vi "utilPlotZeroPole.vi"(3 "a, reverse coefficients":dbl[](array[numeric])=[1.0], 5 "b, forward coefficients":dbl[](array[numeric])) -> (1 "Pole-Zero Plot":cluster{dbl[], dbl[]}[](graph))   [LabVIEW 2016]
doc: "Plot the pole-zero diagram of a filter described by its direct-form \"a\" (reverse) and \"b\" (forward) coefficients."
uses:
  <vilib>/Analysis/1siggen.llb/Ramp Pattern by Samples.vi
  <vilib>/Analysis/polynomials.llb/Remove Zero Coefficients (DBL).vi
  <vilib>/Analysis/polynomials.llb/Polynomial Roots (DBL).vi
  <vilib>/Analysis/NI_AALPro.lvlib
  <vilib>/Analysis/NI_AALBase.lvlib
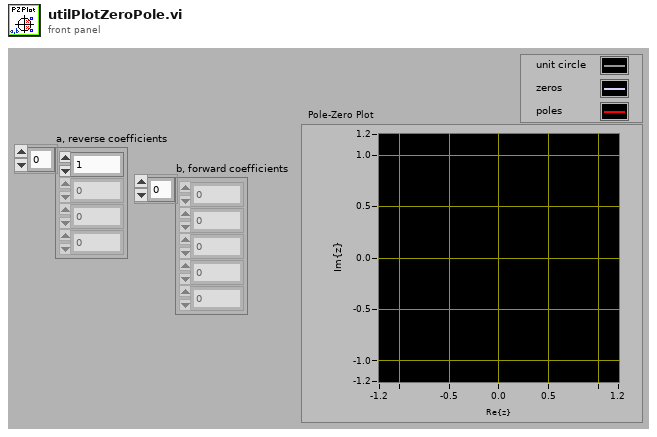
[diagram p1: front panel]
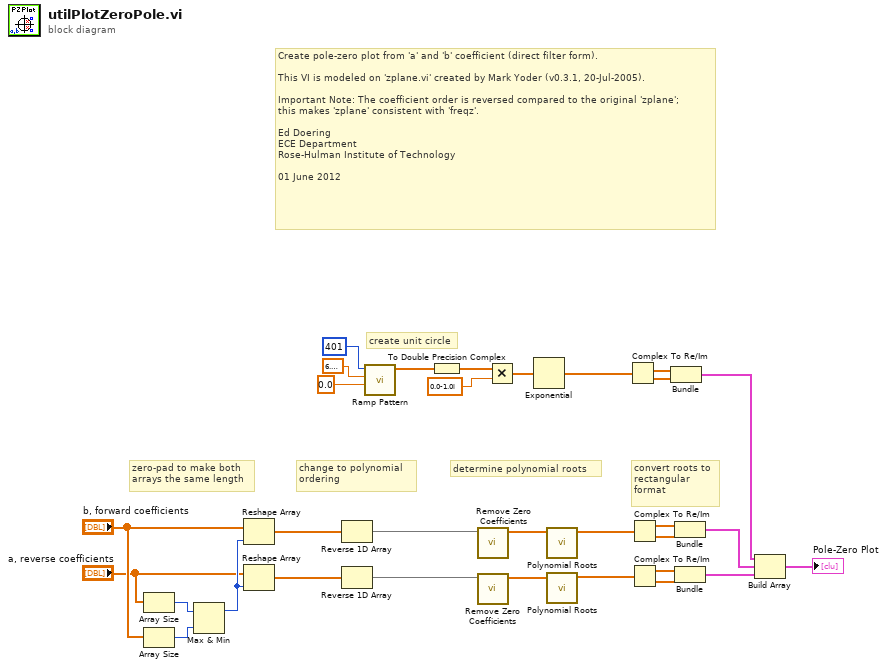
[diagram p0: block diagram]
diagram:
  # "determine polynomial roots"
  # "change to polynomial\nordering"
  # "zero-pad to make both\narrays the same length"
  # "create unit circle"
  # "Create pole-zero plot from 'a' and 'b' coefficient (direct filter form).\n\nThis VI is modeled on 'zplane.vi' created by Mark Yoder (v0.3.1, 20-Jul-2005).\n\nImportant Note: The coefficient order is reversed compared to the original 'zplane';\nthis makes 'zplane' consistent with 'freqz'. \n\nEd Doering\nECE Department\nRose-Hulman Institute of Technology\n\n01 June 2012"
  # "convert roots to\nrectangular \nformat"
  n1 = Array Size(array="a, reverse coefficients") -> (size(s)=w11:i32)
  n2 = Array Size(array="b, forward coefficients") -> (size(s)=w10:i32)
  n3 = Max & Min(x=w11, y=w10) -> (max(x,y)=w9:i32)  [unwired: 1 out]
  n4 = Reshape Array("b, forward coefficients", w9) -> (w6:dbl[])
  n5 = Reshape Array("a, reverse coefficients", w9) -> (w5:dbl[])
  n6 = Reverse 1D Array(array=w6) -> (reversed array=w4:dbl[])
  n7 = Reverse 1D Array(array=w5) -> (reversed array=w3:dbl[])
  n8 = call-poly <vilib>:"Ramp Pattern.vi"("start"=0.0, "end"=6.283185307179586, "samples"=401) -> ("Ramp Pattern"=w19:dbl[])  [unwired: 7 in, 1 out]
  n9 = To Double Precision Complex(1:w19) -> (0:w20:cdb[])
  n10 = call-poly <vilib>:"Remove Zero Coefficients.vi"("P(x) In"=w4) -> ("P(x) Out"=w1:dbl[])  [unwired: 8 in, 2 out]
  n11 = call-poly <vilib>:"Remove Zero Coefficients.vi"("P(x) In"=w3) -> ("P(x) Out"=w2:dbl[])  [unwired: 8 in, 2 out]
  n12 = Multiply(x=w20, y=cdb 0.0-1.0i) -> (x*y=w22:cdb[])
  n13 = Exponential(1:w22) -> (0:w18:cdb[])
  n14 = call-poly <vilib>:"Polynomial Roots.vi"("P(x)"=w1) -> ("Roots"=w13:cdb[])  [unwired: 9 in, 1 out]
  n15 = call-poly <vilib>:"Polynomial Roots.vi"("P(x)"=w2) -> ("Roots"=w12:cdb[])  [unwired: 9 in, 1 out]
  n16 = Complex To Re/Im(x + iy=w18) -> (x=w16:dbl[], y=w17:dbl[])
  n17 = Complex To Re/Im(x + iy=w13) -> (x=w28:dbl[], y=w27:dbl[])
  n18 = Complex To Re/Im(x + iy=w12) -> (x=w26:dbl[], y=w25:dbl[])
  n19 = Bundle(w16, w17) -> (w15:cluster{dbl[], dbl[]})  [unwired: 1 in]
  n20 = Bundle(w28, w27) -> (w30:cluster{dbl[], dbl[]})  [unwired: 1 in]
  n21 = Bundle(w26, w25) -> (w31:cluster{dbl[], dbl[]})  [unwired: 1 in]
  n22 = Build Array(w15, w30, w31) -> (→"Pole-Zero Plot":cluster{dbl[], dbl[]}[])
